vi "TTA_MATLAB_Save_Serial_Number.vi"(8 "error in":errorcluster, 11 "Serial Number":string) -> (0 "error out":errorcluster)   [LabVIEW 2016]
uses:
  TTA_Globals/Test_Environment.vi
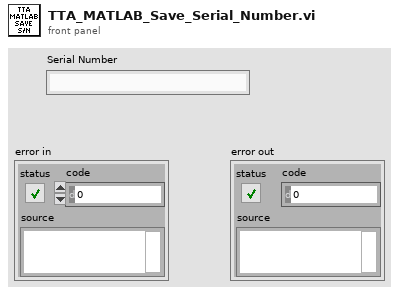
[diagram p1: front panel]
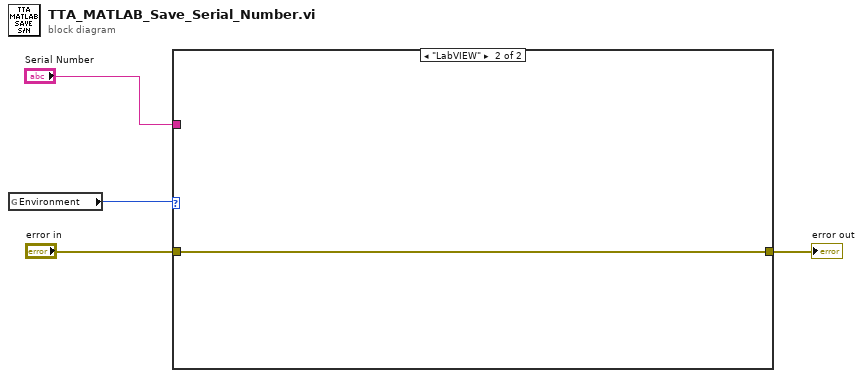
[diagram p0: block diagram]
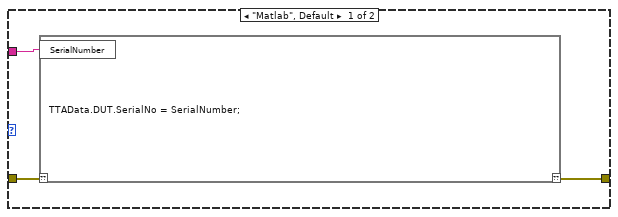
[diagram p2: hidden frame]
diagram:
  n1 = global read "Test_Environment.vi" "Environment"() -> (w1:enum16{"Matlab", "LabVIEW"})
  n2 = case shown="\"LabVIEW\"" w1 {
    tunnel: "error in" -> [w7 w8]
    tunnel: [w6 w8] -> w3
    tunnel: "Serial Number" -> [w5 _]
    frame "Matlab", Default {
      n3 = script code="TTAData.DUT.SerialNo = SerialNumber;"("??"=w7, "SerialNumber"=w5) -> ("??"=w6:errorcluster)
    }
    frame "LabVIEW" {
    }
  }
  "error out" <- w3
